vi "Write Ramp Current.vi"(8 "error in":errorcluster, 10 "Current_Ramp":dbl, 11 "36234A in":refnum<class "36234A.lvclass">) -> (0 "error out":errorcluster, 3 "36234A out":refnum<class "36234A.lvclass">)   [LabVIEW 2019, in "36234A.lvlib" / "36234A.lvclass"]
uses:
  Library/36234A.lvclass
  C:/Users/Public/Documents/Development/builds/Engine/Monitored Actor.lvlibp/Monitored Actor/Monitored Actor/Monitored Actor.lvclass
  C:/Users/Public/Documents/Development/builds/Instruments/Instruments.lvlibp/Library/Instruments.lvclass
  builds/Engine/Monitored Actor.lvlibp/Monitored Actor/Monitored Actor/Read Actor Label.vi
  builds/Instruments/Instruments.lvlibp/Accessors/Generate Warning.vi
  builds/Instruments/PowerSupply.lvlibp/Library/PowerSupply.lvclass
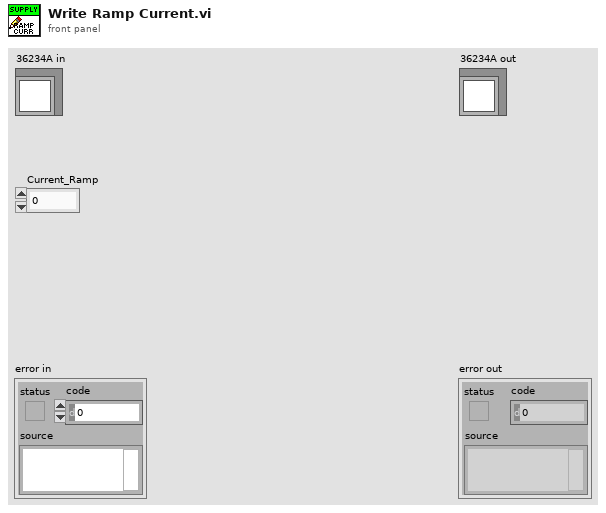
[diagram p1: front panel]
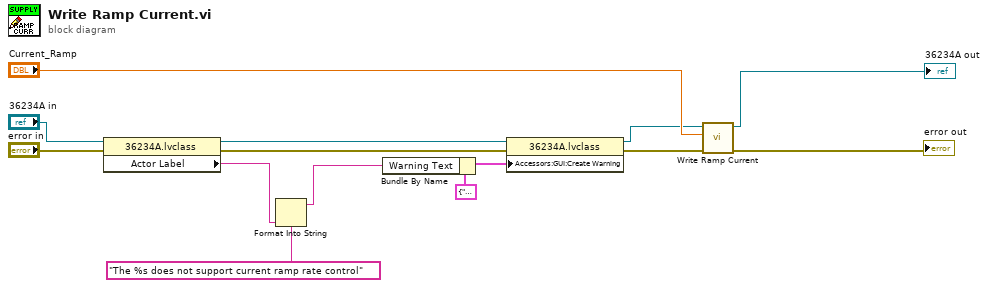
[diagram p0: block diagram]
diagram:
  n1 = property class="36234A.lvclass"(reference="36234A in", error in="error in") -> (reference out=w7:refnum<class "36234A.lvclass">, error out=w10:errorcluster, "Actor Label"=w2:string)
  n2 = Format Into String(format string="The %s does not support current ramp rate control", w2) -> (resulting string=w1:string)  [unwired: 2 in, 1 out]
  n3 = Bundle By Name(cluster=cluster{"Warning Text":string, "code":i32} {"Warning Text"="", "code"=5000008} ("Create Warning"), "Warning Text"=w1) -> (w4:cluster{"Warning Text":string, "code":i32})
  n4 = property class="36234A.lvclass"(reference=w7, error in=w10, "Accessors:GUI:Create Warning"=w4) -> (reference out=w6:refnum<class "36234A.lvclass">, error out=w8:errorcluster)
  n5 = call-parent "Write Ramp Current.vi"("error in"=w8, "Current_Ramp"="Current_Ramp", "PowerSupply in"=w6) -> ("error out"=→"error out":errorcluster, "PowerSupply out"=→"36234A out":refnum<class "36234A.lvclass">)  [unwired: 7 in]
